vi "物流上位机.vi"() -> ()   [LabVIEW 2018]
uses:
  <vilib>/Instr/_visa.llb/VISA Configure Serial Port (Instr).vi
panel:
  in  "停止":bool
  in  "刷新":bool
  out "小车位置":string
  out "小车状态":string
  out "send_flag":bool
  out "运送的物料":string
  out "read buff":string
  in  "发送窗口":string
  in  "send":bool
  out "读取窗口":string
  in  "baud rate (9600)":u64=9600 caption="波特率"
  out "serial":bool
  in  "serial_name":refnum<visa-resource-name> caption="端口"
  in  "serial_open":bool
  in  "停止":bool
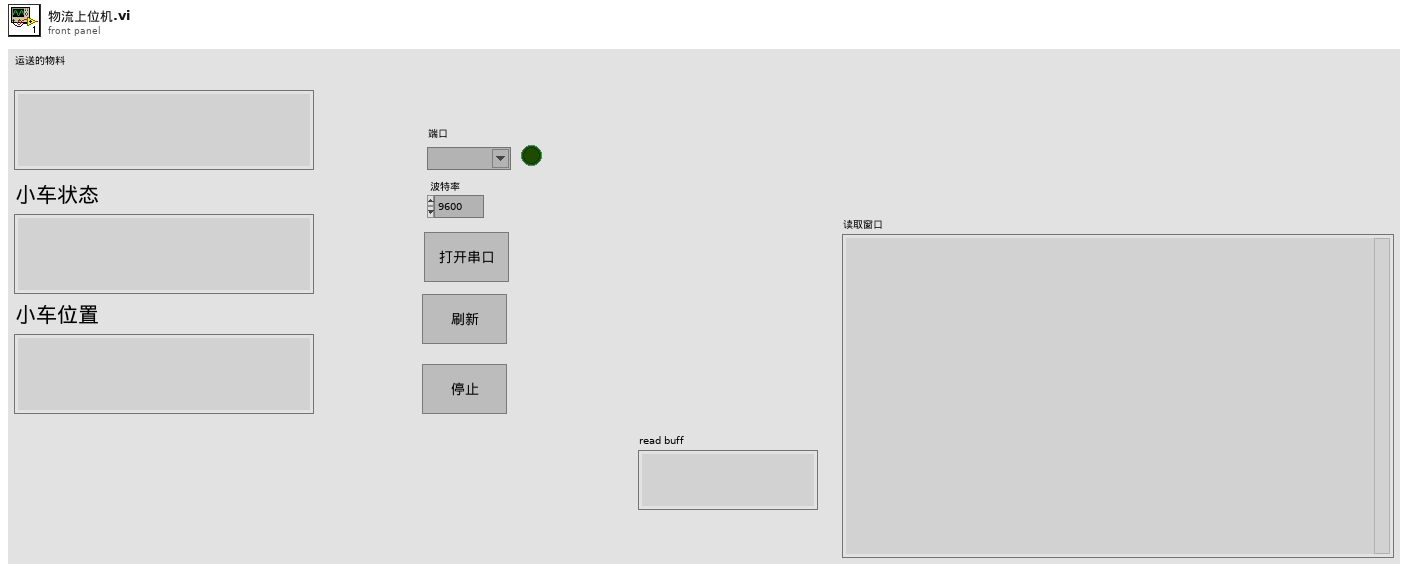
[diagram p1: front panel]
types:
  T1 = typedef "控件.ctl" = enum16{"Init", "send", "Wait", "GatData", "Exit", "deal"}
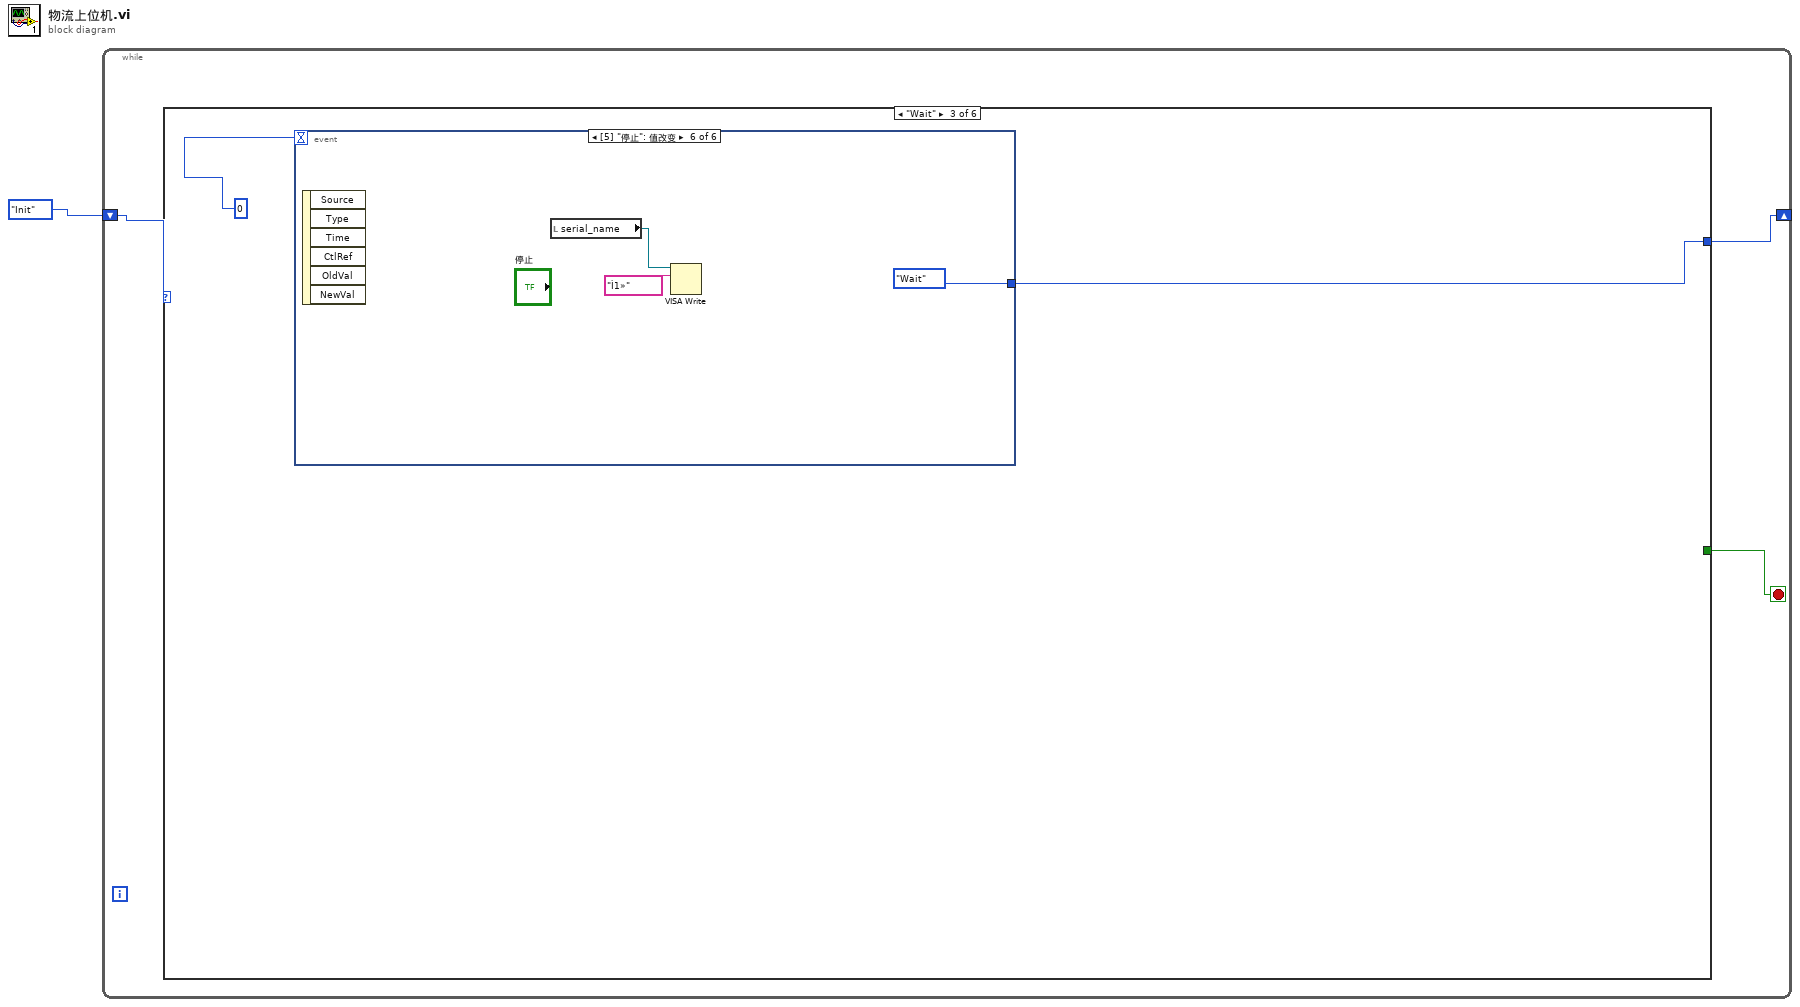
[diagram p0: block diagram]
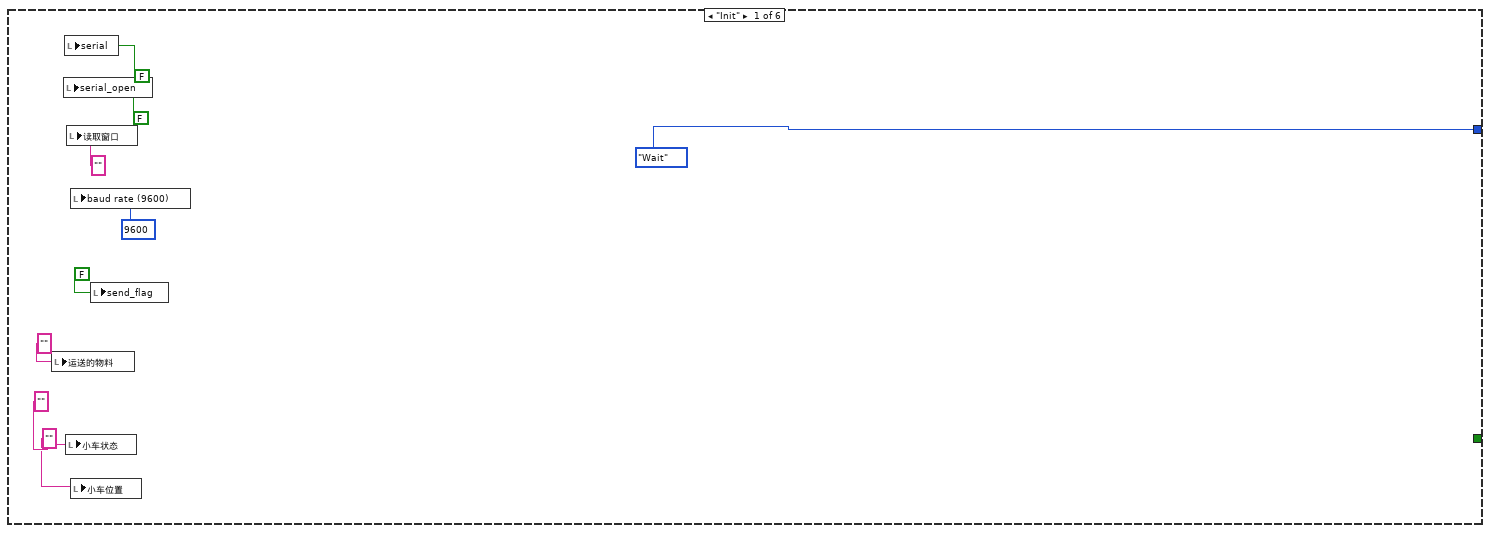
[diagram p2: hidden frame]
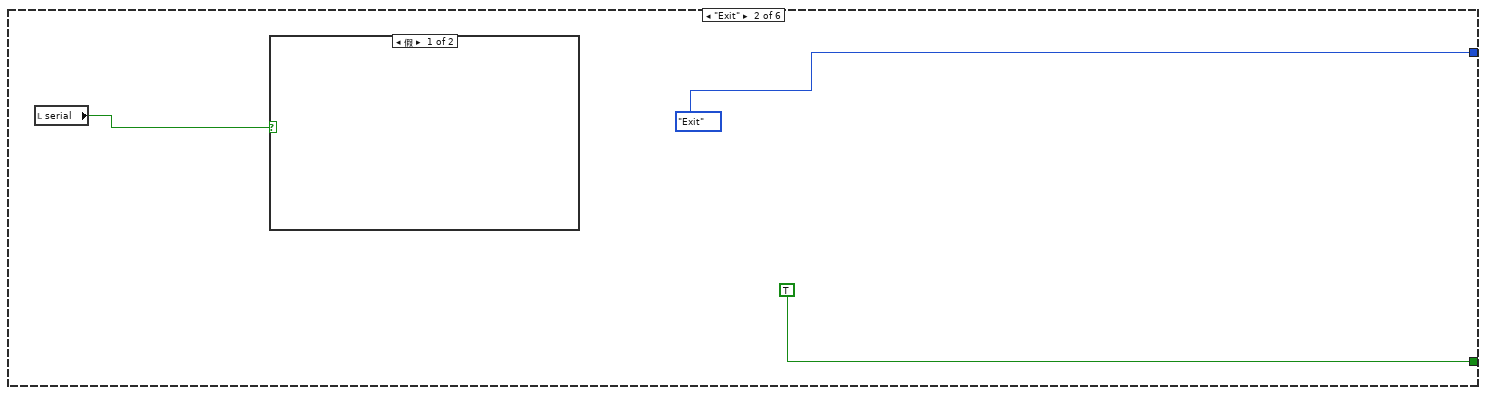
[diagram p3: hidden frame]
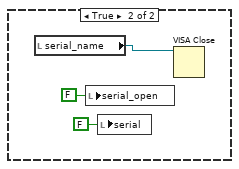
[diagram p4: hidden frame]
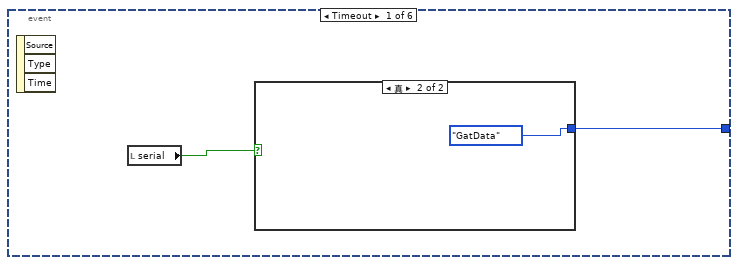
[diagram p5: hidden frame]
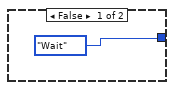
[diagram p6: hidden frame]
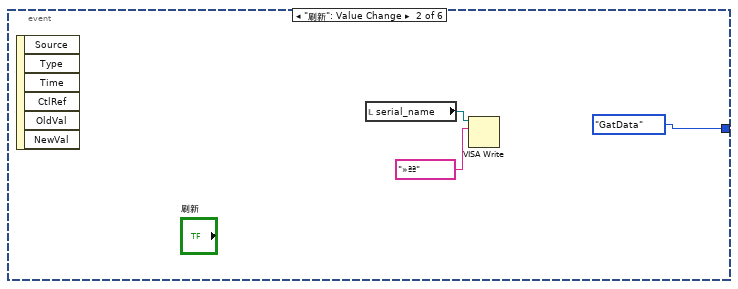
[diagram p7: hidden frame]
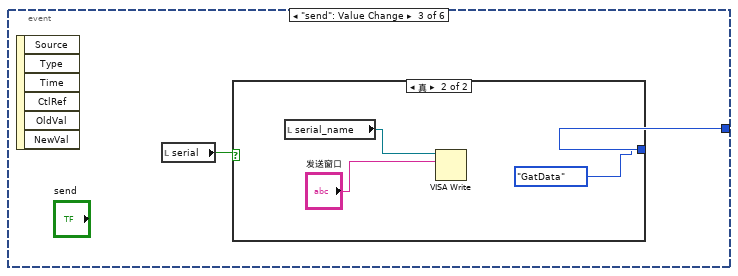
[diagram p8: hidden frame]
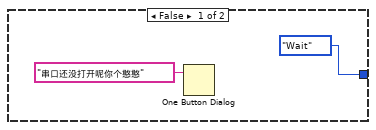
[diagram p9: hidden frame]
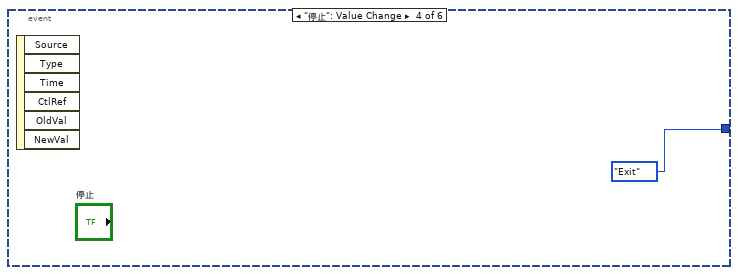
[diagram p10: hidden frame]
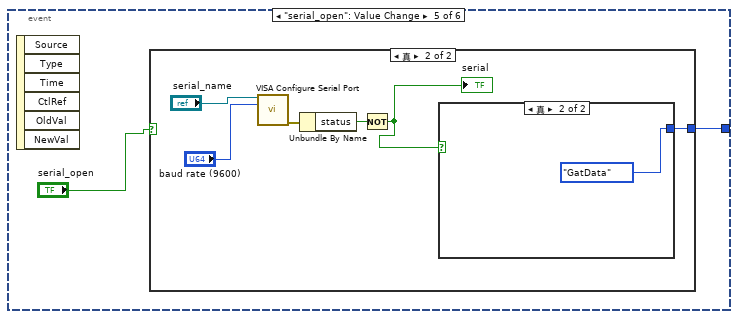
[diagram p11: hidden frame]
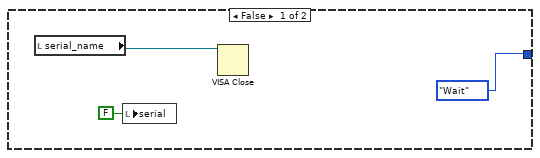
[diagram p12: hidden frame]
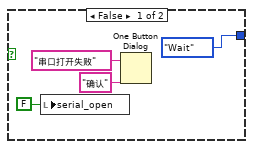
[diagram p13: hidden frame]
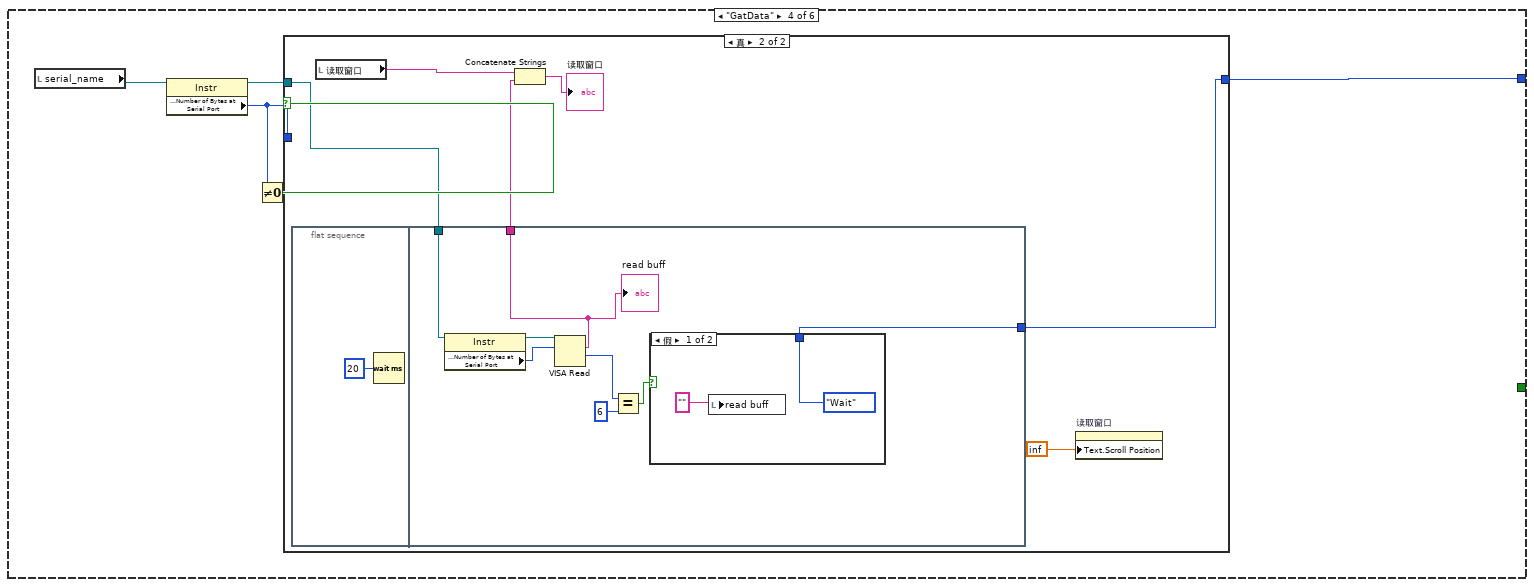
[diagram p14: hidden frame]
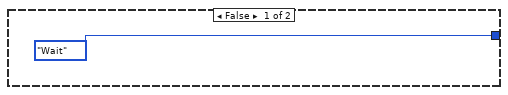
[diagram p15: hidden frame]
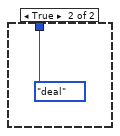
[diagram p16: hidden frame]
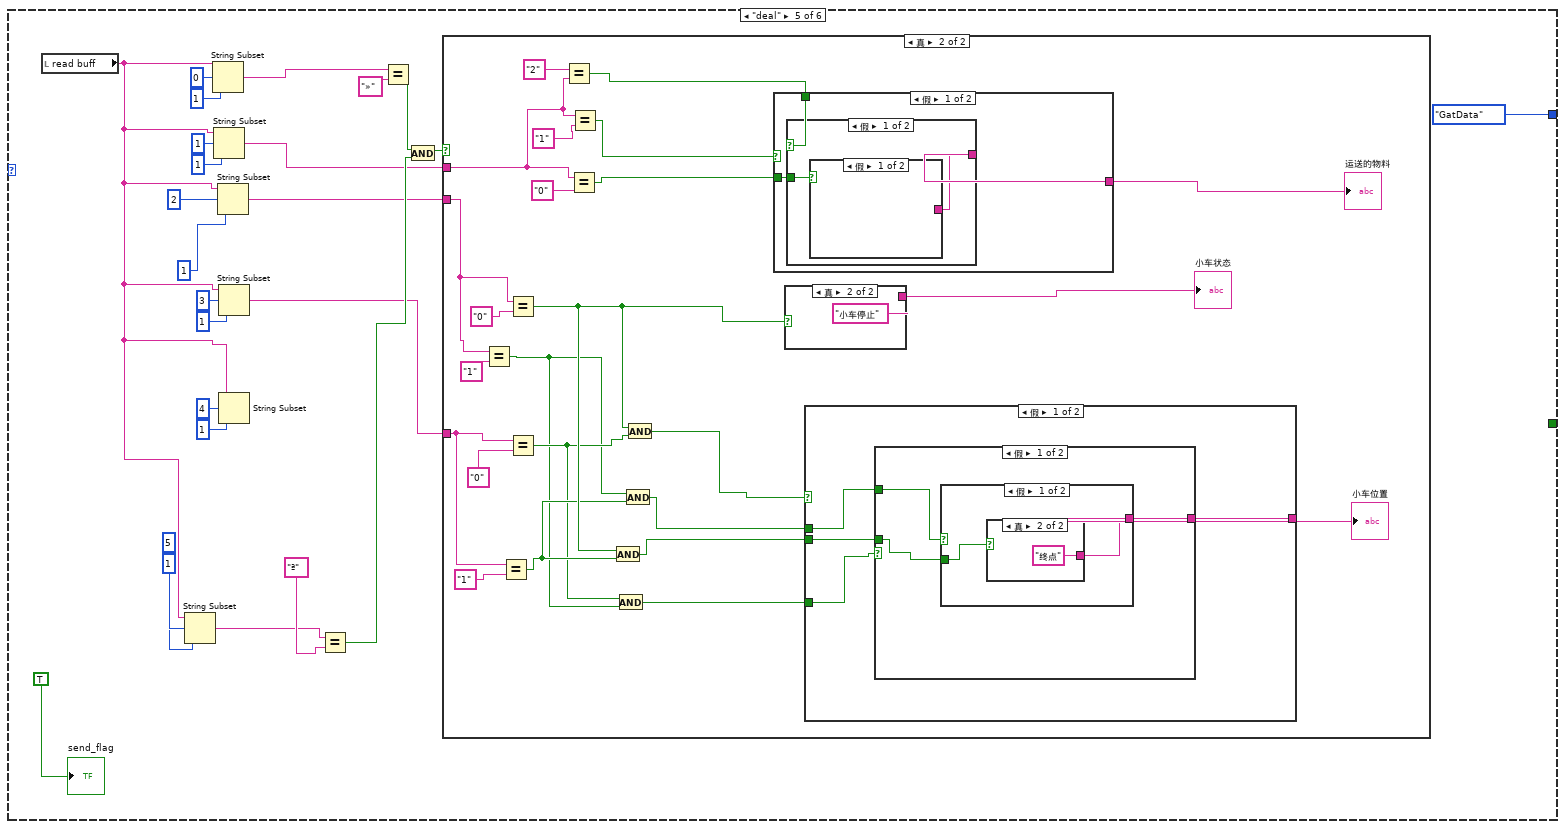
[diagram p17: hidden frame]
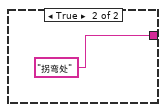
[diagram p20: hidden frame]
diagram:
  n1 = while {
    shift-right: [w3] -> _
    shift-left: 控件."Init" ("枚举") -> [w4]
    stop <- w2 stop-if-true
    n2 = case shown="\"Wait\"" w4 {
      tunnel: [控件."Wait" ("枚举") 控件."Exit" ("枚举") w21 w57 控件."GatData" ("枚举") 控件."Wait" ("枚举")] -> w3
      tunnel: [_ TRUE _ _ _ _] -> w2
      frame "Init" {
        n3 = local write "运送的物料"("" ("子字符串 5")) -> ()
        n4 = local write "serial_open"(FALSE ("serial_open")) -> ()
        n5 = local write "serial"(FALSE ("serial")) -> ()
        n6 = local write "小车状态"("" ("子字符串 5")) -> ()
        n7 = local write "读取窗口"("" ("read buffer")) -> ()
        n8 = local write "baud rate (9600)"(u32 9600 ("baud rate (9600)")) -> ()
        n9 = local write "小车位置"("" ("子字符串 5")) -> ()
        n10 = local write "send_flag"(FALSE ("send_flag")) -> ()
      }
      frame "Exit" {
        n11 = local read "serial"() -> (w15:bool)
        n12 = case shown="假" w15 {
          frame False {
          }
          frame True {
            n13 = local read "serial_name"() -> (w19:refnum<visa-resource-name>)
            n14 = local write "serial_open"(FALSE ("serial_open")) -> ()
            n15 = local write "serial"(FALSE ("serial")) -> ()
            n16 = VISA Close(VISA resource name=w19) -> ()  [unwired: 1 in, 1 out]
          }
        }
      }
      frame "Wait" {
        n17 = event shown="[5] \"停止\": 值改变" {
          selector: _ -> [_ _ _ _ _ _]
          dyn-events: _ -> [_ _ _ _ _ _]
          timeout: 0 -> [_ _ _ _ _ _]
          tunnel: [w22 控件."GatData" ("枚举") w29 控件."Exit" ("枚举") w37 控件."Wait" ("枚举")] -> w21
          event Timeout {
            n18 = event-data() -> ()  [unwired: 1 in, 3 out]
            n19 = local read "serial"() -> (w23:bool)
            n20 = case shown="真" w23 {
              tunnel: [控件."Wait" ("枚举") 控件."GatData" ("枚举")] -> w22
              frame False {
              }
              frame True {
              }
            }
          }
          event "刷新": Value Change {
            n21 = event-data() -> ()  [unwired: 1 in, 6 out]
            n22 = local read "serial_name"() -> (w28:refnum<visa-resource-name>)
            n23 = VISA Write(VISA resource name=w28, write buffer="»ªª" ("数据输入")) -> ()  [unwired: 1 in, 3 out]
          }
          event "send": Value Change {
            n24 = event-data() -> ()  [unwired: 1 in, 6 out]
            n25 = local read "serial"() -> (w30:bool)
            n26 = case shown="真" w30 {
              tunnel: [控件."Wait" ("枚举") 控件."GatData" ("枚举")] -> w29
              frame False {
                n27 = One Button Dialog(message="串口还没打开呢你个憨憨" ("消息")) -> ()  [unwired: 1 in, 1 out]
              }
              frame True {
                n28 = local read "serial_name"() -> (w35:refnum<visa-resource-name>)
                n29 = VISA Write(VISA resource name=w35, write buffer="发送窗口") -> ()  [unwired: 1 in, 3 out]
              }
            }
          }
          event "停止": Value Change {
            n30 = event-data() -> ()  [unwired: 1 in, 6 out]
          }
          event "serial_open": Value Change {
            n31 = event-data() -> ()  [unwired: 1 in, 6 out]
            n32 = case shown="真" "serial_open" {
              tunnel: [控件."Wait" ("枚举") w43] -> w37
              frame False {
                n33 = local read "serial_name"() -> (w41:refnum<visa-resource-name>)
                n34 = local write "serial"(FALSE ("serial")) -> ()
                n35 = VISA Close(VISA resource name=w41) -> ()  [unwired: 1 in, 1 out]
              }
              frame True {
                n36 = call-poly "VISA Configure Serial Port"("VISA resource name"="serial_name", "baud rate (9600)"="baud rate (9600)") -> ("error out"=w46:errorcluster)  [unwired: 12 in, 1 out]
                n37 = Unbundle By Name(w46) -> ("status"=w45:bool)
                n38 = Not(x=w45) -> (.not. x?=w44:bool)
                "serial" <- w44
                n39 = case shown="真" w44 {
                  tunnel: [控件."Wait" ("枚举") 控件."GatData" ("枚举")] -> w43
                  frame False {
                    n40 = local write "serial_open"(FALSE ("serial_open")) -> ()
                    n41 = One Button Dialog(message="串口打开失败" ("消息"), button name ("OK")="确认" ("按钮名称（“确定”）")) -> ()  [unwired: 1 out]
                  }
                  frame True {
                  }
                }
              }
            }
          }
          event "停止": Value Change {
            n42 = event-data() -> ()  [unwired: 1 in, 6 out]
            n43 = local read "serial_name"() -> (w55:refnum<visa-resource-name>)
            n44 = VISA Write(VISA resource name=w55, write buffer="Ì1»") -> ()  [unwired: 1 in, 3 out]
          }
        }
      }
      frame "GatData" {
        n45 = local read "serial_name"() -> (w58:refnum<visa-resource-name>)
        n46 = property on="属性节点" class="Instr"(reference=w58) -> (reference out=w56:refnum<visa-resource-name>, "Serial Settings:Number of Bytes at Serial Port"=w59:u32)  [unwired: 1 in, 1 out]
        n47 = Not Equal To 0?(x=w59) -> (x != 0?=w60:bool)
        n48 = case shown="真" w60 {
          tunnel: w59 -> [_ _]
          tunnel: [控件."Wait" ("枚举") w64] -> w57
          tunnel: w56 -> [_ w63]
          frame False {
          }
          frame True {
            n49 = flat-sequence {
              tunnel: [w74] -> w64
              tunnel: w63 -> [w73]
              tunnel: [w69] -> w62
              frame #0 {
                n50 = Wait (ms)(milliseconds to wait=u32 20 ("等待时间（毫秒）")) -> ()  [unwired: 1 out]
              }
              frame #1 {
                n51 = property on="属性节点" class="Instr"(reference=w73) -> (reference out=w72:refnum<visa-resource-name>, "Serial Settings:Number of Bytes at Serial Port"=w71:u32)  [unwired: 1 in, 1 out]
                n52 = VISA Read(VISA resource name=w72, byte count=w71) -> (read buffer=w69:string, return count=w70:u32)  [unwired: 1 in, 2 out]
                "read buff" <- w69
                n53 = Equal?(x=w70, y=u32 6) -> (x = y?=w76:bool)
                n54 = case shown="假" w76 {
                  tunnel: [控件."Wait" ("枚举") 控件."deal" ("枚举")] -> w74
                  frame False {
                    n55 = local write "read buff"("") -> ()
                  }
                  frame True {
                  }
                }
              }
            }
            n56 = local read "读取窗口"() -> (w66:string)
            n57 = Concatenate Strings(w66, w62) -> (→"读取窗口":string)
            n58 = property on="读取窗口" class="Str"("Text.Scroll Position"=inf) -> ()  [unwired: 2 in, 2 out]
          }
        }
      }
      frame "deal" {
        n59 = local read "read buff"() -> (w85:string)
        n60 = String Subset(string=w85, offset (0)=5 ("偏移量(0)"), length (rest)=1 ("长度（剩余）")) -> (substring=w84:string)
        n61 = String Subset(string=w85, offset (0)=0 ("偏移量(0)"), length (rest)=1 ("长度（剩余）")) -> (substring=w94:string)
        n62 = String Subset(string=w85, offset (0)=1 ("偏移量(0)"), length (rest)=1 ("长度（剩余）")) -> (substring=w91:string)
        n63 = String Subset(string=w85, offset (0)=2 ("偏移量(0)"), length (rest)=1 ("长度（剩余）")) -> (substring=w80:string)
        n64 = String Subset(string=w85, offset (0)=3 ("偏移量(0)"), length (rest)=1 ("长度（剩余）")) -> (substring=w83:string)
        n65 = String Subset(string=w85, offset (0)=4 ("偏移量(0)"), length (rest)=1 ("长度（剩余）")) -> ()  [unwired: 1 out]
        n66 = Equal?(x=w84, y="ª") -> (x = y?=w93:bool)
        n67 = Equal?(x=w94, y="»") -> (x = y?=w96:bool)
        n68 = And(x=w96, y=w93) -> (x .and. y?=w97:bool)
        n69 = case shown="真" w97 {
          tunnel: w91 -> [_ w107]
          tunnel: w83 -> [_ w118]
          tunnel: w80 -> [_ w120]
          frame False {
          }
          frame True {
            n70 = Equal?(x=w120, y="1") -> (x = y?=w110:bool)
            n71 = Equal?(x=w118, y="1") -> (x = y?=w112:bool)
            n72 = Equal?(x=w120, y="0") -> (x = y?=w114:bool)
            n73 = Equal?(x=w118, y="0") -> (x = y?=w111:bool)
            n74 = Equal?(x="2" ("y"), y=w107) -> (x = y?=w116:bool)
            n75 = Equal?(x=w107, y="0") -> (x = y?=w105:bool)
            n76 = Equal?(x=w107, y="1") -> (x = y?=w122:bool)
            n77 = And(x=w114, y=w112) -> (x .and. y?=w108:bool)
            n78 = And(x=w111, y=w110) -> (x .and. y?=w109:bool)
            n79 = And(x=w110, y=w112) -> (x .and. y?=w113:bool)
            n80 = And(x=w114, y=w111) -> (x .and. y?=w115:bool)
            n81 = case shown="假" w122 {
              tunnel: [w145 "螺帽" ("子字符串 4")] -> w123
              tunnel: w116 -> [w146 _]
              tunnel: w105 -> [w144 _]
              frame False {
                n82 = case shown="假" w146 {
                  tunnel: [w147 "铜柱" ("子字符串 4")] -> w145
                  tunnel: w144 -> [w148 _]
                  frame False {
                    n83 = case shown="假" w148 {
                      tunnel: [_ "获取到货物信息中" ("子字符串 4")] -> w147
                      frame False {
                      }
                      frame True {
                      }
                    }
                  }
                  frame True {
                  }
                }
              }
              frame True {
              }
            }
            "运送的物料" <- w123
            n84 = case shown="真" w114 {
              tunnel: ["运行中" ("子字符串 4") "小车停止" ("子字符串 4")] -> w127
              frame False {
              }
              frame True {
              }
            }
            "小车状态" <- w127
            n85 = case shown="假" w115 {
              tunnel: [w131 "起点位置" ("子字符串 4")] -> w125
              tunnel: w113 -> [w129 _]
              tunnel: w109 -> [w132 _]
              tunnel: w108 -> [w130 _]
              frame False {
                n86 = case shown="假" w132 {
                  tunnel: [w135 "直线运行" ("子字符串 4")] -> w131
                  tunnel: w130 -> [w134 _]
                  tunnel: w129 -> [w133 _]
                  frame False {
                    n87 = case shown="假" w133 {
                      tunnel: [w137 "拐弯处" ("子字符串 4")] -> w135
                      tunnel: w134 -> [w136 _]
                      frame False {
                        n88 = case shown="真" w136 {
                          tunnel: [_ "终点" ("子字符串 4")] -> w137
                          frame False {
                          }
                          frame True {
                          }
                        }
                      }
                      frame True {
                      }
                    }
                  }
                  frame True {
                  }
                }
              }
              frame True {
              }
            }
            "小车位置" <- w125
          }
        }
        "send_flag" <- TRUE ("布尔")
      }
      frame "send" {
      }
    }
  }
